vi "recondense_set_Monitor_Values.vi"(1 "System Monitor Variables (in)":T1) -> (0 "System Monitor Variables (out)":T1)   [LabVIEW 2019]
uses:
  Global/Global Variables/System Monitor Cluster.ctl
  Global/Global Variables/Data_Display_global.vi
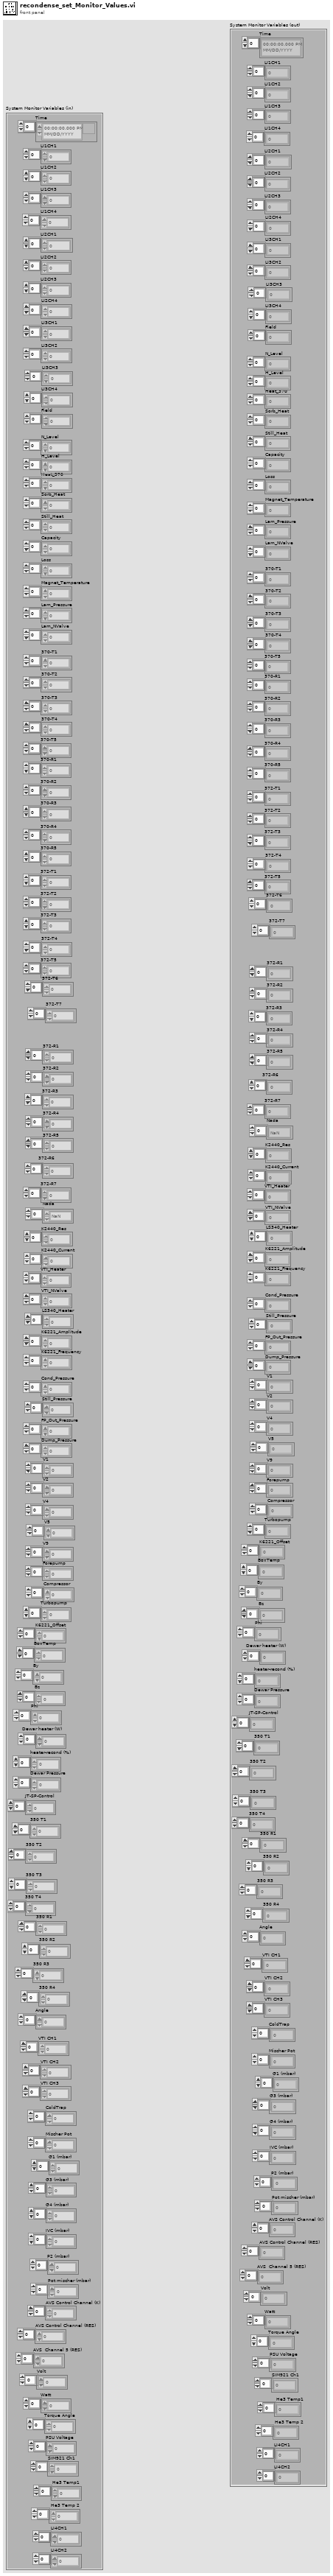
[diagram p1: front panel]
types:
  T1 = typedef "System Monitor Cluster.ctl" = cluster{"Time":timestamp[], "LI1CH1":dbl[], "LI1CH2":dbl[], "LI2CH1":dbl[], "LI2CH2":dbl[], "LI3CH1":dbl[], "LI3CH2":dbl[], "Field":dbl[], "N_Level":dbl[], "H_Level":dbl[], "Heat_370":dbl[], "Sorb_Heat":dbl[], "Still_Heat":dbl[], "Capacity":dbl[], "Loss":dbl[], "Magnet_Temperature":dbl[], "Lam_Pressure":dbl[], "Lam_NValve":dbl[], "370-T1":dbl[], "370-T2":dbl[], "370-T3":dbl[], "370-T4":dbl[], "370-T5":dbl[], "370-R1":dbl[], "370-R2":dbl[], "370-R3":dbl[], "370-R4":dbl[], "370-R5":dbl[], "372-T1":dbl[], "372-T2":dbl[], "372-T3":dbl[], "372-T4":dbl[], "372-T5":dbl[], "372-T6":dbl[], "372-R1":dbl[], "372-R2":dbl[], "372-R3":dbl[], "372-R4":dbl[], "372-R5":dbl[], "372-R6":dbl[], "Nada":dbl[], "K2440_Res":dbl[], "K2440_Current":dbl[], "VTI_Heater":dbl[], "VTI_NValve":dbl[], "LS340_Heater":dbl[], "K6221_Amplitude":dbl[], "K6221_Frequency":dbl[], "Cond_Pressure":dbl[], "Still_Pressure":dbl[], "FP_Out_Pressure":dbl[], "Dump_Pressure":dbl[], "V1":dbl[], "V2":dbl[], "V4":dbl[], "V5":dbl[], "V9":dbl[], "Forepump":dbl[], "Compressor":dbl[], "K6221_Offset":dbl[], "BoxTemp":dbl[], "By":dbl[], "Bz":dbl[], "Phi":dbl[], "heater-recond (%)":dbl[], "Dewar Pressure ":dbl[], "JT-SP-Control":dbl[], "350 T1":dbl[], "350 T2":dbl[], "350 T3":dbl[], "350 T4":dbl[], "350 R1":dbl[], "350 R2":dbl[], "350 R3":dbl[], "350 R4":dbl[], "Angle":dbl[], "VTI CH1":dbl[], "VTI CH2":dbl[], "VTI CH3":dbl[], "ColdTrap":dbl[], "Mischer Pot":dbl[], "G1 (mbar)":dbl[], "G3 (mbar) ":dbl[], "G4 (mbar)":dbl[], "IVC (mbar)":dbl[], "P2 (mbar) ":dbl[], "Pot mischer (mbar)":dbl[], "AVS Control Channel (K)":dbl[], "AVS Control Channel (RES)":dbl[], "AVS  Channel 5 (RES) ":dbl[], "LI3CH3":dbl[], "LI3CH4":dbl[], "LI1CH3":dbl[], "LI1CH4":dbl[], "LI2CH3":dbl[], "LI2CH4":dbl[], "Volt":dbl[], "Watt":dbl[], "Torque Angle":dbl[], "Dewar heater (W)":dbl[], "PSU Voltage":dbl[], "Turbopump":dbl[], "372-R7":dbl[], "372-T7":dbl[], "SIM921 Ch1":dbl[], " He3 Temp1":dbl[], " He3 Temp 2":dbl[], "LI4CH1":dbl[], "LI4CH2":dbl[]}
  T2 = typedef "BorowskiMonitor.ctl" = cluster{"Sorb Temp":dbl, "1K Temp":dbl, "He3 Temp 1":dbl, "He3 Temp2":dbl, "Recondense Complete?":bool, "Sorb Heater Auto?":bool, "Sorb Heater On?":bool, "Sorb Setpoint":dbl, "Sorb Heater %":dbl, "Begin Recondense":bool, "He3-Pot Setpoint":dbl, "He3-Pot Heater %":dbl, "He3 Heater Auto?":bool, "He3 Heater On?":bool, "He3-Pot Temperature Control":bool}
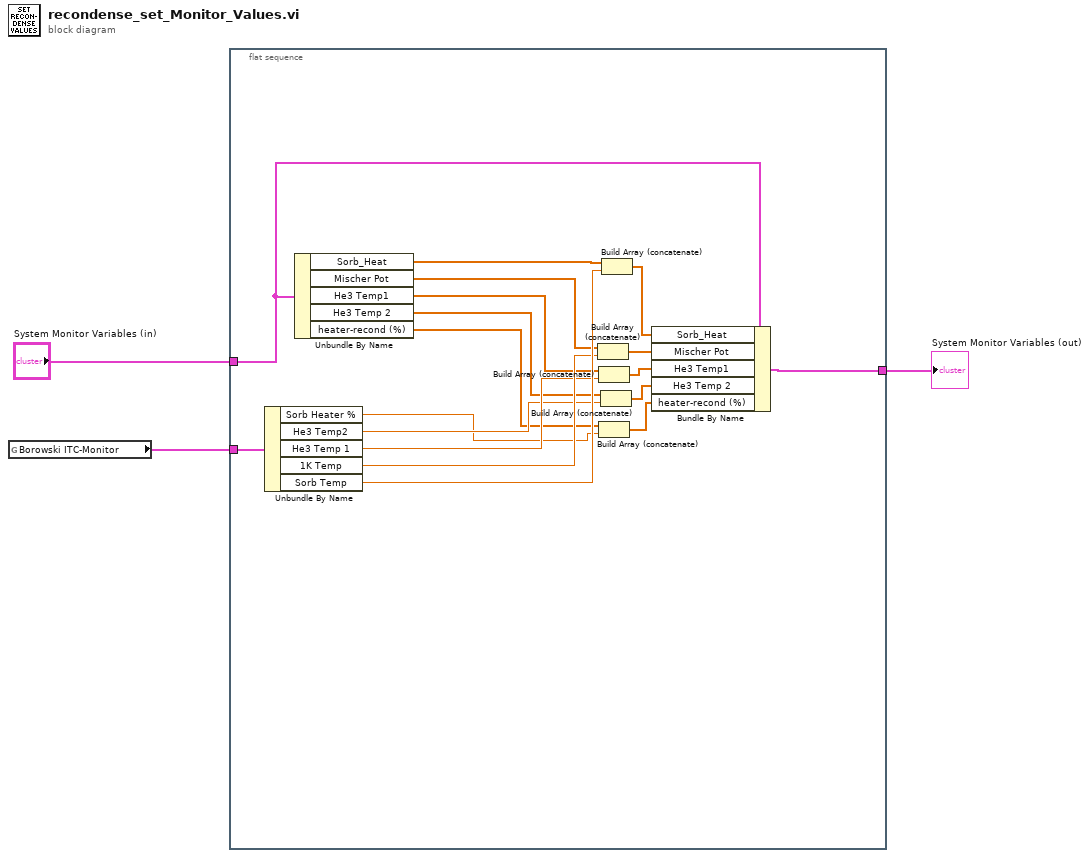
[diagram p0: block diagram]
diagram:
  n1 = global read "Data_Display_global.vi" "Borowski ITC-Monitor"() -> (w2:T2)
  n2 = flat-sequence {
    tunnel: "System Monitor Variables (in)" -> [w20]
    tunnel: w2 -> [w21]
    tunnel: [w19] -> w1
    frame #0 {
      n3 = Unbundle By Name(w21) -> ("Sorb Heater %"=w4:dbl, "He3 Temp2"=w7:dbl, "He3 Temp 1"=w8:dbl, "1K Temp"=w10:dbl, "Sorb Temp"=w17:dbl)
      n4 = Unbundle By Name(w20) -> ("Sorb_Heat"=w18:dbl[], "Mischer Pot"=w11:dbl[], "He3 Temp1"=w9:dbl[], "He3 Temp 2"=w6:dbl[], "heater-recond (%)"=w5:dbl[])
      n5 = Build Array (concatenate)(w11, w10) -> (w15:dbl[])
      n6 = Build Array (concatenate)(w9, w8) -> (w14:dbl[])
      n7 = Build Array (concatenate)(w5, w4) -> (w12:dbl[])
      n8 = Build Array (concatenate)(w6, w7) -> (w13:dbl[])
      n9 = Build Array (concatenate)(w18, w17) -> (w16:dbl[])
      n10 = Bundle By Name(cluster=w20, "Sorb_Heat"=w16, "Mischer Pot"=w15, "He3 Temp1"=w14, "He3 Temp 2"=w13, "heater-recond (%)"=w12) -> (w19:T1)
    }
  }
  "System Monitor Variables (out)" <- w1
